vi "Apply SA.vi"(7 "Perturbation Method":T1, 8 "error in (no error)":errorcluster, 9 "Scheduler.lvclass":refnum<class "Scheduler.lvclass">, 10 "GA.lvclass":refnum<class "GA.lvclass">, 11 "OSSP_Problem in":refnum<class "OSSP_Problem.lvclass">) -> (0 "error out":errorcluster, 1 "Scheduler.lvclass Out":refnum<class "Scheduler.lvclass">, 2 "GA out":refnum<class "GA.lvclass">, 3 "OSSP_Problem out":refnum<class "OSSP_Problem.lvclass">)   [LabVIEW 2013]
uses:
  Classes/GA.lvclass
  Classes/OSSP_Problem.lvclass
  Classes/SA_Class/Controls/Perturbation Method.ctl
  Classes/Scheduler.lvclass
  Classes/GA.lvclass/GA.ctl
  Classes/SA.lvclass
  SA/Controls/States_SA.ctl
  Classes/SA_Class/Controls/CoolingScheme.ctl
  Classes/SA.lvclass/SA.ctl
  Classes/SA_Class/Controls/Solution_SA.ctl
  Classes/Scheduler.lvclass/Scheduler.ctl
  Classes/OSSP_Problem.lvclass/OSSP_Problem.ctl
  Classes/Scheduler_Class/NonDelay Scheduler/Non Delay Scheduler Engine.vi
  Classes/OSSP_Problem_Class/Getters/Read Number of Jobs.vi
  Classes/OSSP_Problem_Class/Getters/Read Number of Machines.vi
  Classes/OSSP_Problem_Class/Getters/Read Processing Times.vi
  Calcualte General Tardiness.vi
  Classes/OSSP_Problem_Class/Getters/Read Due Dates.vi
  Classes/Scheduler_Class/Giffler Thompson Active Schedule Engine.vi
  Classes/Scheduler_Class/Prins FIFO Scheduler Methods and Controls/Methods/Calculate Makespan (Prins FIFO Engine).vi
  Classes/Scheduler_Class/Prins FIFO Scheduler Methods and Controls/Methods/Calculate Tardiness (Prins FIFO Engine).vi
  Classes/Scheduler_Class/Modified GT Active Scheduler/GT Active Scheduler wSubset4Tardiness.vi
  Classes/Scheduler_Class/Getters/Read Lambda.vi
  Classes/Scheduler_Class/Getters/Read Operation Selection Rule.vi
  Classes/Scheduler_Class/Getters/Read Scheduler.vi
  Remove Duplicates In Array.vi
  Classes/Scheduler_Class/Operation to Machine Job Tuple.vi
  Classes/Scheduler_Class/Prins FIFO Scheduler Methods and Controls/Prins FIFO Scheduler.vi
  Classes/Scheduler_Class/Prins FIFO Scheduler Methods and Controls/Methods/Calculate Final Completion Times of Jobs.vi
  Classes/Scheduler_Class/Prins FIFO Scheduler Methods and Controls/Methods/Reorder Schedule(Prins FIFO) based on Start Times.vi
  Classes/Scheduler_Class/Modified GT Active Scheduler/GT Find Subset of Operations.vi
  Classes/Scheduler_Class/Modified GT Active Scheduler/Select Operation to Schedule Based on Rule.vi
  Classes/Scheduler_Class/Prins FIFO Scheduler Methods and Controls/Methods/UpdateMachineGaps.vi
  Classes/Scheduler_Class/Prins FIFO Scheduler Methods and Controls/Methods/UpdateJobGaps.vi
  Classes/Scheduler_Class/Prins FIFO Scheduler Methods and Controls/Methods/Find Intersecting Gaps.vi
  Classes/Scheduler_Class/GT Algorithm Find M_ok and J_ok.vi
  Classes/Scheduler_Class/Prins FIFO Scheduler Methods and Controls/Methods/Transform to Plain Job and Machine Gaps Array.vi
  Classes/Scheduler_Class/Semiactive Scheduler/Semi Active Scheduler Engine.vi
panel:
  out "Thermometer":dbl(slide) scale=0.0..100.0
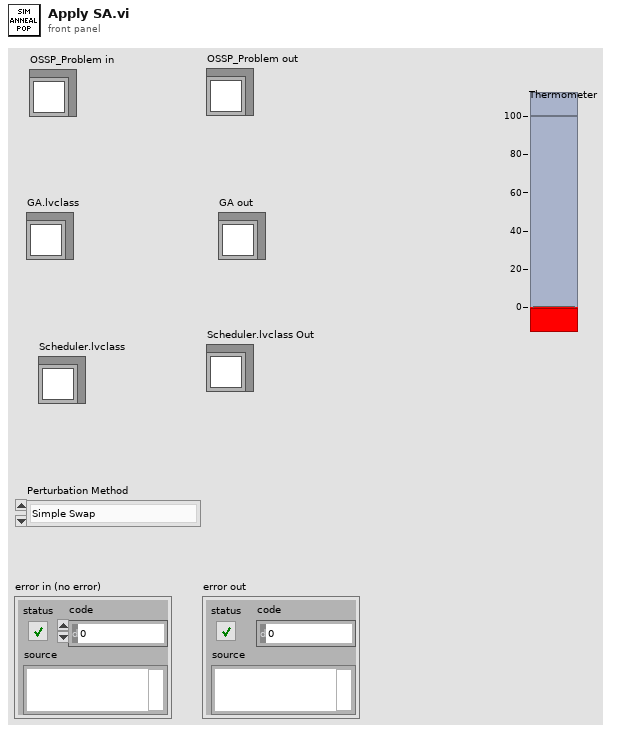
[diagram p1: front panel]
types:
  T1 = typedef "SA.lvclass/Perturbation Method.ctl" = enum16{"Simple Swap", "Insert", "NonRedundantSwap", "Job Order Swap", "Machine Order Swap", "Machine&Job Order Swap", "Critical Path Swap"}
  T2 = typedef "Solution_GA.ctl" = cluster{"Schedule":u16[], "Fitness":u16, "Fitness Valid?":bool}
  T3 = typedef "States_SA.ctl" = enum16{"Init", "Read Problem", "Sort Problem", "Generate and Evaluate Current Solution", "Perturb Cur Solution and Eval New Solution", "Make Decision", "Keep Track of Best Solution", "Cool", "Output Final Solution", "Stop"}
  T4 = typedef "SA.lvclass/CoolingScheme.ctl" = enum16{"Linear", "Geometric"}
  T5 = typedef "SA.lvclass/Solution_SA.ctl" = cluster{"Schedule":u16[], "Fitness":u16}
  T6 = typedef "Objective.ctl" = enum16{"Makespan", "Total Tardiness"}
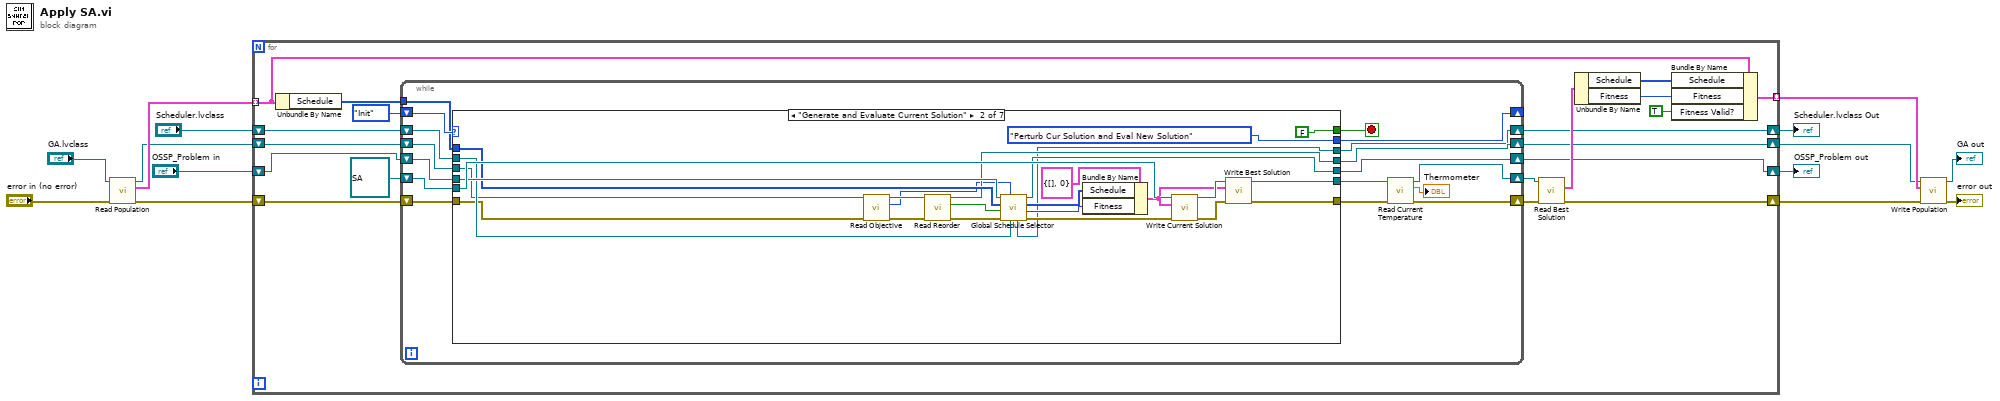
[diagram p0: block diagram]
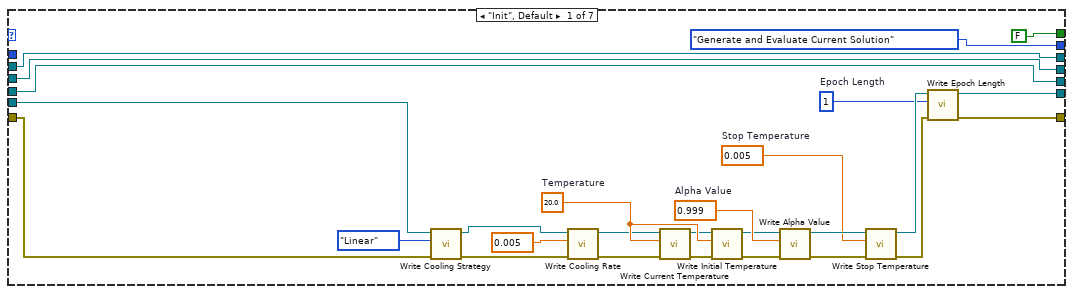
[diagram p2: hidden frame]
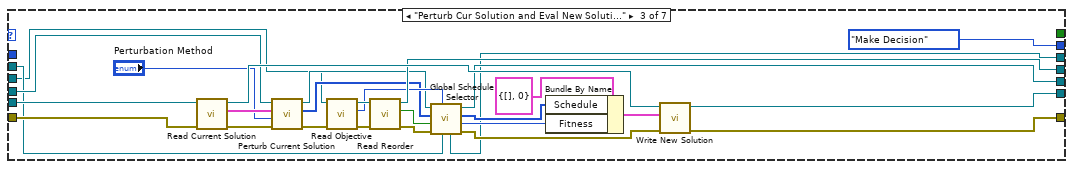
[diagram p3: hidden frame]
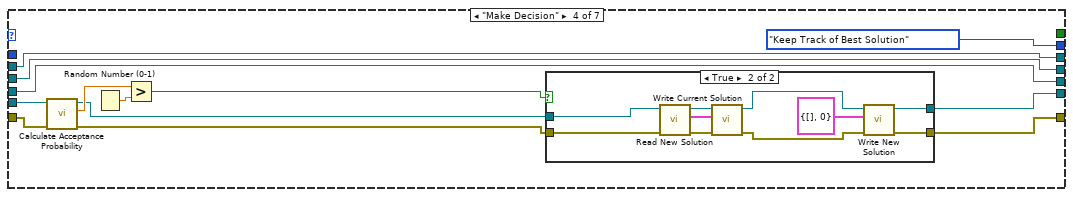
[diagram p4: hidden frame]
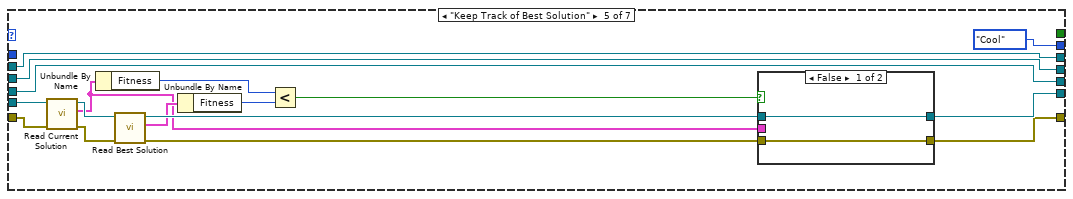
[diagram p6: hidden frame]
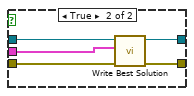
[diagram p7: hidden frame]
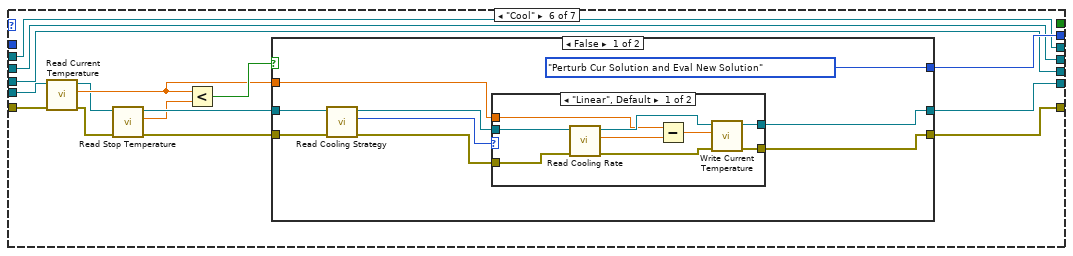
[diagram p8: hidden frame]
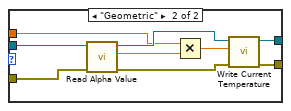
[diagram p9: hidden frame]
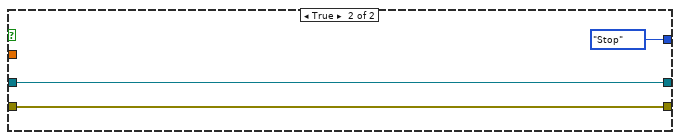
[diagram p10: hidden frame]
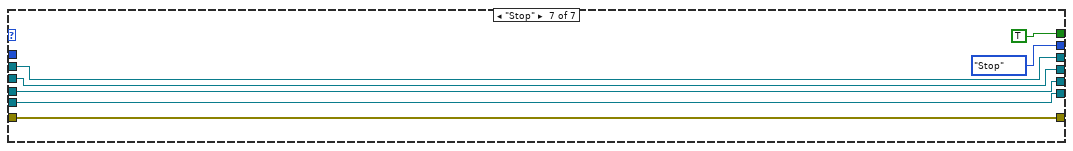
[diagram p11: hidden frame]
diagram:
  n1 = call "Read Population.vi"("error in (no error)"="error in (no error)", "GA in"="GA.lvclass") -> ("error out"=w7:errorcluster, "Population"=w9:T2[], "GA out"=w4:refnum<class "GA.lvclass">)  [unwired: 7 in]
  n2 = for {
    tunnel: w9 -> [w29] mode=indexing
    tunnel: [w24] -> w8 mode=indexing
    shift-right: [w23] -> w6
    shift-left: w7 -> [w20]
    shift-right: [w21] -> w5
    shift-left: w4 -> [w19]
    shift-right: [w17] -> w3
    shift-left: "OSSP_Problem in" -> [w18]
    shift-right: [w15] -> w1
    shift-left: "Scheduler.lvclass" -> [w16]
    n3 = Unbundle By Name(w29) -> ("Schedule"=w33:u16[])
    n4 = while {
      tunnel: w33 -> [w48]
      shift-right: [w47] -> _
      shift-left: States_SA."Init" ("States") -> [w50]
      shift-right: [w42] -> w30
      shift-left: refnum<class "SA.lvclass"> refnum ("SA.lvclass") -> [w49]
      shift-right: [w38] -> w17
      shift-left: w18 -> [w40]
      shift-right: [w39] -> w22
      shift-left: w20 -> [w45]
      shift-right: [w36] -> w21
      shift-left: w19 -> [w37]
      shift-right: [w34] -> w15
      shift-left: w16 -> [w35]
      stop <- w46 stop-if-true
      n5 = case shown="\"Generate and Evaluate Current Solution\"" w50 {
        tunnel: w49 -> [w74 w102 w130 w143 w172 w194 w230]
        tunnel: w48 -> [_ w90 _ _ _ _ _]
        tunnel: [w58 w97 w126 w142 w171 w191 w230] -> w43
        tunnel: [States_SA."Generate and Evaluate Current Solution" ("States") States_SA."Perturb Cur Solution and Eval New Solution" ("States") States_SA."Make Decision" ("States") States_SA."Keep Track of Best Solution" States_SA."Cool" w190 States_SA."Stop"] -> w47
        tunnel: [FALSE FALSE _ _ _ _ TRUE] -> w46
        tunnel: [w56 w94 w124 w136 w159 w188 w228] -> w44
        tunnel: w45 -> [w70 w79 w120 w135 w160 w189 w228]
        tunnel: w40 -> [w53 w93 w111 w133 w158 w182 w227]
        tunnel: [w53 w92 w117 w133 w158 w182 w227] -> w38
        tunnel: w37 -> [w52 w78 w104 w132 w157 w181 w226]
        tunnel: [w52 w84 w115 w132 w157 w181 w226] -> w36
        tunnel: w35 -> [w51 w81 w106 w131 w156 w180 w225]
        tunnel: [w51 w80 w103 w131 w156 w180 w225] -> w34
        frame "Init", Default {
          w55 = u8 1  # Epoch Length
          w61 = 0.005  # Stop Temperature
          w77 = 0.999  # Alpha Value
          w67 = 20.0  # Temperature
          n6 = call "Write Cooling Strategy.vi"("error in (no error)"=w70, "Cooling Strategy"=CoolingScheme."Linear", "SA in"=w74) -> ("error out"=w71:errorcluster, "SA out"=w72:refnum<class "SA.lvclass">)  [unwired: 7 in]
          n7 = call "Write Cooling Rate.vi"("error in (no error)"=w71, "Cooling Rate"=0.005, "SA in"=w72) -> ("error out"=w69:errorcluster, "SA out"=w54:refnum<class "SA.lvclass">)  [unwired: 7 in]
          n8 = call "Write Current Temperature.vi"("error in (no error)"=w69, "Temperature"=w67, "SA in"=w54) -> ("error out"=w66:errorcluster, "SA out"=w64:refnum<class "SA.lvclass">)  [unwired: 7 in]
          n9 = call "Write Initial Temperature.vi"("error in (no error)"=w66, "Initial Temperature"=w67, "SA in"=w64) -> ("error out"=w65:errorcluster, "SA out"=w63:refnum<class "SA.lvclass">)  [unwired: 7 in]
          n10 = call "Write Alpha Value.vi"("error in (no error)"=w65, "Alpha Value"=w77, "SA in"=w63) -> ("error out"=w60:errorcluster, "SA out"=w62:refnum<class "SA.lvclass">)  [unwired: 7 in]
          n11 = call "Write Stop Temperature.vi"("error in (no error)"=w60, "Stop Temperature"=w61, "SA in"=w62) -> ("error out"=w57:errorcluster, "SA out"=w59:refnum<class "SA.lvclass">)  [unwired: 7 in]
          n12 = call "Write Epoch Length.vi"("error in (no error)"=w57, "Epoch Length"=w55, "SA in"=w59) -> ("error out"=w56:errorcluster, "SA out"=w58:refnum<class "SA.lvclass">)  [unwired: 7 in]
        }
        frame "Generate and Evaluate Current Solution" {
          n13 = call "Read Objective .vi"("error in (no error)"=w79, "GA in"=w78) -> ("error out"=w87:errorcluster, "Objective"=w83:T6, "GA out"=w85:refnum<class "GA.lvclass">)  [unwired: 7 in]
          n14 = call "Read Reorder.vi"("error in (no error)"=w87, "GA in"=w85) -> ("error out"=w86:errorcluster, "Reorder"=w82:bool, "GA out"=w84:refnum<class "GA.lvclass">)  [unwired: 7 in]
          n15 = call "Global Schedule Selector.vi"("Scheduler In"=w81, "Objective"=w83, "error in (no error)"=w86, "Reorder?"=w82, "Schedule in"=w90, "OSSP_Problem in"=w93) -> ("error out"=w91:errorcluster, "Total Tardiness or Makespan (U16)"=w88:u16, "Schedule out"=w89:u16[], "OSSP_Problem out"=w92:refnum<class "OSSP_Problem.lvclass">, "Scheduler out"=w80:refnum<class "Scheduler.lvclass">)  [unwired: 1 in]
          n16 = Bundle By Name(cluster=T5 {"Schedule"=[], "Fitness"=0} ("Solution"), "Schedule"=w89, "Fitness"=w88) -> (w96:T5)
          n17 = call "Write Current Solution.vi"("error in (no error)"=w91, "Solution"=w96, "SA in"=w102) -> ("error out"=w95:errorcluster, "SA out"=w98:refnum<class "SA.lvclass">)  [unwired: 7 in]
          n18 = call "Write Best Solution.vi"("error in (no error)"=w95, "Solution"=w96, "SA in"=w98) -> ("error out"=w94:errorcluster, "SA out"=w97:refnum<class "SA.lvclass">)  [unwired: 7 in]
        }
        frame "Perturb Cur Solution and Eval New Solution" {
          n19 = call "Read Current Solution.vi"("error in (no error)"=w120, "SA in"=w130) -> ("error out"=w123:errorcluster, "Solution"=w109:T5, "SA out"=w129:refnum<class "SA.lvclass">)  [unwired: 7 in]
          n20 = call "Perturb Current Solution.vi"("error in (no error)"=w123, "Perturbation Method"="Perturbation Method", "Solution"=w109, "OSSP_Problem In"=w111) -> ("error out"=w105:errorcluster, "Perturbed Schedule"=w107:u16[], "OSSP_Problem out"=w110:refnum<class "OSSP_Problem.lvclass">)  [unwired: 5 in]
          n21 = call "Read Objective .vi"("error in (no error)"=w105, "GA in"=w104) -> ("error out"=w119:errorcluster, "Objective"=w114:T6, "GA out"=w121:refnum<class "GA.lvclass">)  [unwired: 7 in]
          n22 = call "Read Reorder.vi"("error in (no error)"=w119, "GA in"=w121) -> ("error out"=w122:errorcluster, "Reorder"=w116:bool, "GA out"=w115:refnum<class "GA.lvclass">)  [unwired: 7 in]
          n23 = call "Global Schedule Selector.vi"("Scheduler In"=w106, "Objective"=w114, "error in (no error)"=w122, "Reorder?"=w116, "Schedule in"=w107, "OSSP_Problem in"=w110) -> ("error out"=w118:errorcluster, "Total Tardiness or Makespan (U16)"=w112:u16, "Schedule out"=w113:u16[], "OSSP_Problem out"=w117:refnum<class "OSSP_Problem.lvclass">, "Scheduler out"=w103:refnum<class "Scheduler.lvclass">)  [unwired: 1 in]
          n24 = Bundle By Name(cluster=T5 {"Schedule"=[], "Fitness"=0} ("Solution"), "Schedule"=w113, "Fitness"=w112) -> (w127:T5)
          n25 = call "Write New Solution.vi"("error in (no error)"=w118, "Solution"=w127, "SA in"=w129) -> ("error out"=w124:errorcluster, "SA out"=w126:refnum<class "SA.lvclass">)  [unwired: 7 in]
        }
        frame "Make Decision" {
          n26 = call "Calculate Acceptance Probability.vi"("error in (no error)"=w135, "SA in"=w143) -> ("error out"=w134:errorcluster, "Acceptance Probability"=w140:dbl, "SA out"=w137:refnum<class "SA.lvclass">)  [unwired: 7 in]
          n27 = Random Number (0-1)() -> (number: 0 to 1=w139:dbl)
          n28 = Greater?(x=w140, y=w139) -> (0:w138:bool)
          n29 = case shown="True" w138 {
            tunnel: w137 -> [w145 w155]
            tunnel: [w145 w149] -> w142
            tunnel: w134 -> [w144 w148]
            tunnel: [w144 w146] -> w136
            frame False {
            }
            frame True {
              n30 = call "Read New Solution.vi"("error in (no error)"=w148, "SA in"=w155) -> ("error out"=w154:errorcluster, "Solution"=w152:T5, "SA out"=w153:refnum<class "SA.lvclass">)  [unwired: 7 in]
              n31 = call "Write Current Solution.vi"("error in (no error)"=w154, "Solution"=w152, "SA in"=w153) -> ("error out"=w150:errorcluster, "SA out"=w151:refnum<class "SA.lvclass">)  [unwired: 7 in]
              n32 = call "Write New Solution.vi"("error in (no error)"=w150, "Solution"=T5 {"Schedule"=[], "Fitness"=0}, "SA in"=w151) -> ("error out"=w146:errorcluster, "SA out"=w149:refnum<class "SA.lvclass">)  [unwired: 7 in]
            }
          }
        }
        frame "Keep Track of Best Solution" {
          n33 = call "Read Current Solution.vi"("error in (no error)"=w160, "SA in"=w172) -> ("error out"=w162:errorcluster, "Solution"=w164:T5, "SA out"=w170:refnum<class "SA.lvclass">)  [unwired: 7 in]
          n34 = Unbundle By Name(w164) -> ("Fitness"=w168:u16)
          n35 = call "Read Best Solution.vi"("error in (no error)"=w162, "SA in"=w170) -> ("error out"=w161:errorcluster, "Solution"=w167:T5, "SA out"=w169:refnum<class "SA.lvclass">)  [unwired: 7 in]
          n36 = Unbundle By Name(w167) -> ("Fitness"=w166:u16)
          n37 = Less?(x=w168, y=w166) -> (x < y?=w165:bool)
          n38 = case shown="False" w165 {
            tunnel: w169 -> [w174 w179]
            tunnel: [w174 w178] -> w171
            tunnel: w164 -> [_ w177]
            tunnel: w161 -> [w173 w176]
            tunnel: [w173 w175] -> w159
            frame False {
            }
            frame True {
              n39 = call "Write Best Solution.vi"("error in (no error)"=w176, "Solution"=w177, "SA in"=w179) -> ("error out"=w175:errorcluster, "SA out"=w178:refnum<class "SA.lvclass">)  [unwired: 7 in]
            }
          }
        }
        frame "Cool" {
          n40 = call "Read Current Temperature.vi"("error in (no error)"=w189, "SA in"=w194) -> ("error out"=w187:errorcluster, "Temperature"=w192:dbl, "SA out"=w185:refnum<class "SA.lvclass">)  [unwired: 7 in]
          n41 = call "Read Stop Temperature.vi"("error in (no error)"=w187, "SA in"=w185) -> ("error out"=w186:errorcluster, "Stop Temperature"=w183:dbl, "SA out"=w184:refnum<class "SA.lvclass">)  [unwired: 7 in]
          n42 = Less?(x=w192, y=w183) -> (x < y?=w193:bool)
          n43 = case shown="False" w193 {
            tunnel: [States_SA."Perturb Cur Solution and Eval New Solution" ("f") States_SA."Stop"] -> w190
            tunnel: w184 -> [w199 w223]
            tunnel: [w202 w223] -> w191
            tunnel: w192 -> [w201 _]
            tunnel: w186 -> [w197 w222]
            tunnel: [w200 w222] -> w188
            frame False {
              n44 = call "Read Cooling Strategy.vi"("error in (no error)"=w197, "SA in"=w199) -> ("error out"=w196:errorcluster, "Cooling Strategy"=w195:T4, "SA out"=w198:refnum<class "SA.lvclass">)  [unwired: 7 in]
              n45 = case shown="\"Linear\", Default" w195 {
                tunnel: [w207 w221] -> w202
                tunnel: w198 -> [w211 w220]
                tunnel: w201 -> [w206 w214]
                tunnel: w196 -> [w212 w216]
                tunnel: [w208 w215] -> w200
                frame "Linear", Default {
                  n46 = call "Read Cooling Rate.vi"("error in (no error)"=w212, "SA in"=w211) -> ("error out"=w209:errorcluster, "Cooling Rate"=w205:dbl, "SA out"=w210:refnum<class "SA.lvclass">)  [unwired: 7 in]
                  n47 = Subtract(x=w206, y=w205) -> (x-y=w204:dbl)
                  n48 = call "Write Current Temperature.vi"("error in (no error)"=w209, "Temperature"=w204, "SA in"=w210) -> ("error out"=w208:errorcluster, "SA out"=w207:refnum<class "SA.lvclass">)  [unwired: 7 in]
                }
                frame "Geometric" {
                  n49 = call "Read Alpha Value.vi"("error in (no error)"=w216, "SA in"=w220) -> ("error out"=w218:errorcluster, "Alpha Value"=w213:dbl, "SA out"=w219:refnum<class "SA.lvclass">)  [unwired: 7 in]
                  n50 = Multiply(x=w214, y=w213) -> (x*y=w217:dbl)
                  n51 = call "Write Current Temperature.vi"("error in (no error)"=w218, "Temperature"=w217, "SA in"=w219) -> ("error out"=w215:errorcluster, "SA out"=w221:refnum<class "SA.lvclass">)  [unwired: 7 in]
                }
              }
            }
            frame True {
            }
          }
        }
        frame "Stop" {
        }
      }
      n52 = call "Read Current Temperature.vi"("error in (no error)"=w44, "SA in"=w43) -> ("error out"=w39:errorcluster, "Temperature"=→"Thermometer":dbl, "SA out"=w42:refnum<class "SA.lvclass">)  [unwired: 7 in]
    }
    n53 = call "Read Best Solution.vi"("error in (no error)"=w22, "SA in"=w30) -> ("error out"=w23:errorcluster, "Solution"=w28:T5)  [unwired: 7 in, 1 out]
    n54 = Unbundle By Name(w28) -> ("Schedule"=w27:u16[], "Fitness"=w26:u16)
    n55 = Bundle By Name(cluster=w29, "Schedule"=w27, "Fitness"=w26, "Fitness Valid?"=TRUE) -> (w24:T2)
  }
  "OSSP_Problem out" <- w3
  "Scheduler.lvclass Out" <- w1
  n56 = call "Write Population.vi"("error in (no error)"=w6, "Population"=w8, "GA in"=w5) -> ("error out"=→"error out":errorcluster, "GA out"=→"GA out":refnum<class "GA.lvclass">)  [unwired: 7 in]
